vi "FormatSimpleMessage.vi"(8 "error in":errorcluster, 11 "cmd":string) -> (0 "error out":errorcluster, 3 "JSON string":string)   [LabVIEW 2014, in "Raspberry Pi Compatible Compiler for LabVIEW.lvlib" / "RasPiDownloader.lvlib"]
uses:
  RasPiDownloader.lvlib
  SimpleCommandTD.ctl
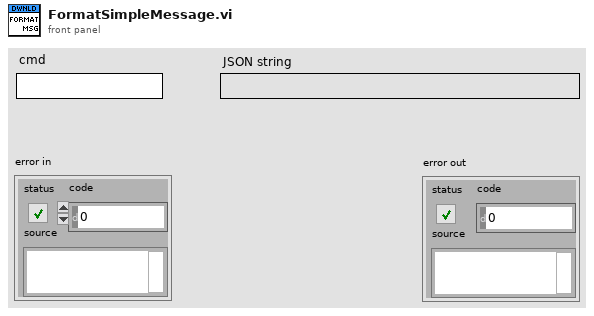
[diagram p1: front panel]
types:
  T1 = typedef "Raspberry Pi Compatible Compiler for LabVIEW.lvlib/RasPiDownloader.lvlib/SimpleCommandTD.ctl" = cluster{"cmd":string}
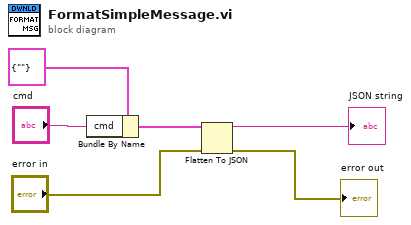
[diagram p0: block diagram]
diagram:
  n1 = Bundle By Name(cluster=T1 {"cmd"=""} ("message"), "cmd"="cmd") -> (w4:T1)
  n2 = Flatten To JSON(anything=w4, error in (no error)="error in") -> (JSON string=→"JSON string":string, 11:→"error out":errorcluster)  [unwired: 1 in]
